vi "DSF.Shared.Configuration.Framework.Create From String.vi"(8 "error in (no error)":errorcluster, 10 "String":string) -> (0 "error out":errorcluster, 3 "Framework Configuration":refnum<class "DSF.Shared.Configuration.Framework.lvclass">)   [LabVIEW 2016, in "DSF.Shared.lvlib" / "DSF.Shared.Configuration.Framework.lvclass"]
uses:
  DSF.Shared.Configuration.Framework.lvclass
  C:/Git/SourceTree/DSF/Source/Shared/Classes/Configuration/DSF.Shared.Configuration.lvclass
  Configuration/DSF.Shared.Configuration.lvclass
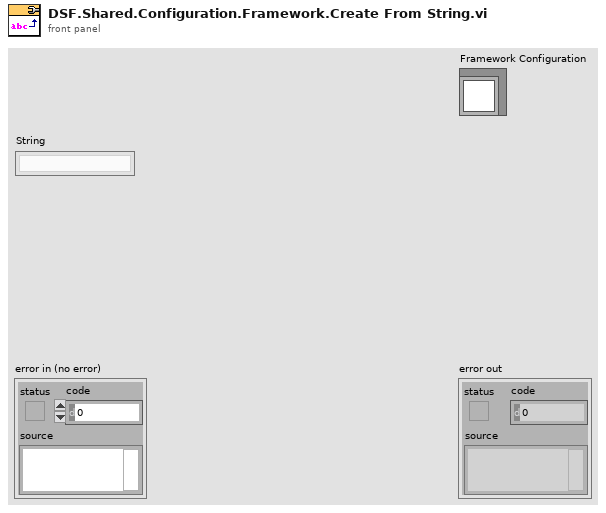
[diagram p1: front panel]
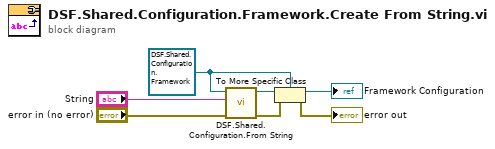
[diagram p0: block diagram]
diagram:
  w6 = refnum<class "DSF.Shared.Configuration.Framework.lvclass"> refnum ("Transfer Configuration out")
  n1 = call "DSF.Shared.Configuration.From String.vi"("error in (no error)"="error in (no error)", "String"="String", "Configuration in"=w6) -> ("error out"=w5:errorcluster, "Configuration out"=w7:refnum<class "DSF.Shared.Configuration.lvclass">)  [unwired: 7 in]
  n2 = To More Specific Class(target class=w6, reference=w7, error in=w5) -> (specific class reference=→"Framework Configuration":refnum<class "DSF.Shared.Configuration.Framework.lvclass">, error out=→"error out":errorcluster)
